vi "Get flattened data.vi"(8 "error in (no error)":errorcluster, 11 "DatagridElement in":refnum<class "DatagridElement.lvclass">) -> (0 "error out":errorcluster, 2 "Flattened data":u8[](array[numeric]), 3 "DatagridElement out":refnum<class "DatagridElement.lvclass">)   [LabVIEW 2018, in "D Datagrid Library.lvlib" / "DatagridElement.lvclass"]
uses:
  DatagridElement.lvclass
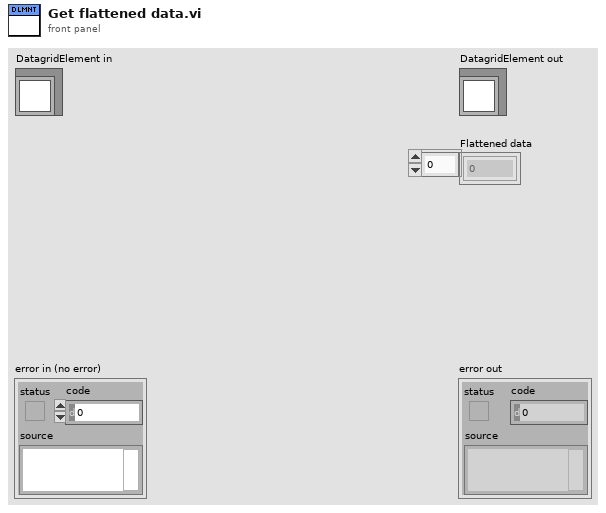
[diagram p1: front panel]
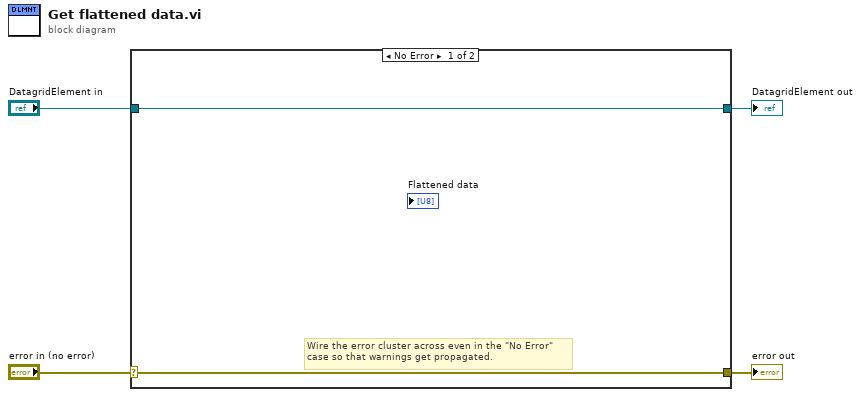
[diagram p0: block diagram]
diagram:
  n1 = case shown="No Error" "error in (no error)" {
    selector: "error in (no error)" -> [w5 w8]
    tunnel: [w5 w8] -> w3
    tunnel: [w6 w7] -> w1
    tunnel: "DatagridElement in" -> [w6 w7]
    frame No Error {
      # "Wire the error cluster across even in the \"No Error\"\ncase so that warnings get propagated."
    }
    frame Error {
    }
  }
  "error out" <- w3
  "DatagridElement out" <- w1
